vi "AplyDAQpars1.vi"(5 "AcqTimeIn":dbl) -> (1 "t1-t0":dbl, 3 "Idxs":i32[](array[numeric]))   [LabVIEW 2010]
uses:
  70user.lib/TheSigTab.vi
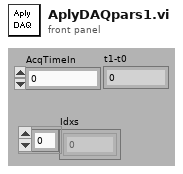
[diagram p1: front panel]
types:
  T1 = cluster{"Status":bool, "ViErrorNumber":u32, "ViName":string, "ViErrorString":string, "CinName":string, "CinErrorString":string}
  T2 = cluster{"s_Type":u16, "FIFO":u16, "IrqStep":u16, "Pages":u16, "AutoInit":u16, "dRate":dbl, "dKadr":dbl, "dScale":dbl, "Rate":u16, "Kadr":u16, "Scale":u16, "FPDelay":u16, "SynchroType":u16, "SynchroSensitivity":u16, "SynchroMode":u16, "AdChannel":u16, "AdPorog":u16, "NCh":u16, "Chn":i32[], "IrqEna":u16, "AdcEna":u16}
  T3 = cluster{"DllVersion":u32, "InterfaceType":u32, "InterfaceInstance":u32, "ModuleHandle":u32, "ReadBuffersParsArray":cluster{"Buffer":i16[], "ReadOv":u32, "ReadEvent":u32}[], "WriteBuffersParsArray":cluster{"Buffer":i16[], "WriteOv":u32, "WriteEvent":u32}[]}
  T4 = cluster{"VirtualSlot":u16, "ModuleName":string, "SerialNumber":string, "UsbSpeed":u8, "AvrVersion":string, "ModuleRevision":string, "DspType":string, "IsDacPresented":bool, "DspLoading":bool, "DspVersion":string, "DspClockout":u32, "AdcOffsetCoef":sgl[], "AdcScaleCoef":sgl[], "DacOffsetCoef":sgl[], "DacScaleCoef":sgl[]}
  T5 = cluster{"size":u16, "InputEnabled":bool, "CorrectionEnabled":bool, "InputClockSource":u16, "InputType":u16, "SynchroType":u16, "SynchroAdType":u16, "SynchroAdMode":u16, "SynchroAdChannel":u16, "SynchroAdPorog":i16, "ChannelsQuantity":u16, "ControlTable":u16[], "InputFifoBaseAddress":u16, "InputFifoLength":u16, "InputRate":dbl, "InterKadrDelay":dbl, "ChannelRate":dbl, "AdcOffsetCoefArray":dbl[], "AdcScaleCoefArray":dbl[], "BuffersLengthArray":u32[]}
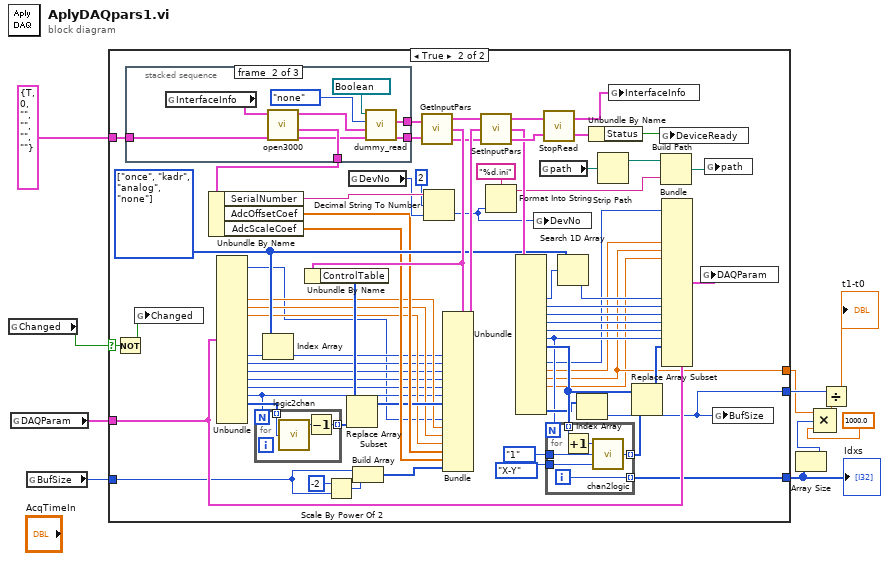
[diagram p0: block diagram]
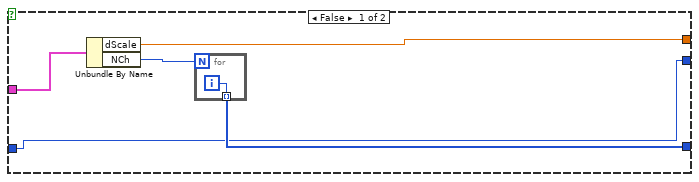
[diagram p2: hidden frame]
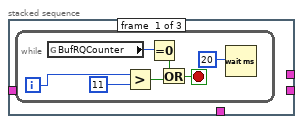
[diagram p3: hidden frame]
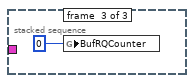
[diagram p4: hidden frame]
diagram:
  n1 = global read "TheSigTab.vi" "Changed"() -> (w11:bool)
  n2 = global read "TheSigTab.vi" "DAQParam"() -> (w10:T2)
  n3 = global read "TheSigTab.vi" "BufSize"() -> (w8:u32)
  n4 = case shown="True" w11 {
    selector: w11 -> [_ w66]
    tunnel: [w14 w46] -> w7
    tunnel: w10 -> [w16 w64]
    tunnel: T1 {"Status"=TRUE, "ViErrorNumber"=0, "ViName"="", "ViErrorString"="", "CinName"="", "CinErrorString"=""} ("ViStatusOut") -> [_ w60]
    tunnel: w8 -> [w12 w45]
    tunnel: [w12 w44] -> w6
    tunnel: [w13 w19] -> w5
    frame False {
      n5 = Unbundle By Name(w16) -> ("dScale"=w13:dbl, "NCh"=w15:u16)
      n6 = for {
        N: w15 -> [_]
        tunnel: [w17] -> w14 mode=indexing
        i -> [w17]
      }
    }
    frame True {
      w69 = enum16{"none", "once", "kadr", "analog"}[] [enum."once", enum."kadr", enum."analog", enum."none"] items=["none", "once", "kadr", "analog"]
      n7 = Not(x=w66) -> (.not. x?=w65:bool)
      n8 = stacked-sequence {
        tunnel: w60 -> [_ w101 _]
        tunnel: [_ w95 _] -> w59
        tunnel: [_ w96 _] -> w58
        tunnel: [_ w99 _] -> w57
        frame #0 {
          n9 = while {
            i -> [w91]
            stop <- w87 stop-if-true
            n10 = global read "TheSigTab.vi" "BufRQCounter"() -> (w92:i32)
            n11 = Greater?(x=w91, y=11) -> (0:w89:bool)
            n12 = Equal To 0?(x=w92) -> (x = 0?=w88:bool)
            n13 = Or(x=w88, y=w89) -> (x .or. y?=w87:bool)
            n14 = Wait (ms)(milliseconds to wait=u32 20) -> ()  [unwired: 1 out]
          }
        }
        frame #1 {
          n15 = global read "TheSigTab.vi" "InterfaceInfo"() -> (w100:T3)
          n16 = call "open3000.vi"("ViInfo"=w101, "InterfaceInfo"=w100) -> ("ViInfoOut"=w98:T1, "ModuleInfo"=w99:T4, "InterfaceInfoOut"=w97:T3)  [unwired: 3 in]
          n17 = call "dummy_read.vi"("ViStatusOut 2"=w98, "InterfaceInfoOut 2"=w97, "SyncType3000"=enum16{"none", "TTL", "TTL_kadr", "analog"}."none", "Ctrl Reference"=refnum<vi> refnum) -> ("ViStatusOut"=w96:T1, "InterfaceInfoOut"=w95:T3)  [unwired: 2 in]
        }
        frame #2 {
          n18 = global write "TheSigTab.vi" "BufRQCounter"(0 ("BufRQCounter")) -> ()
        }
      }
      n19 = global write "TheSigTab.vi" "Changed"(w65) -> ()
      n20 = Unbundle By Name(w57) -> ("SerialNumber"=w56:string, "AdcOffsetCoef"=w41:sgl[], "AdcScaleCoef"=w42:sgl[])
      n21 = Unbundle(w64) -> ("FIFO"=w22:u16, "dRate"=w37:dbl, "dKadr"=w36:dbl, "dScale"=w35:dbl, "SynchroType"=w71:u16, "SynchroSensitivity"=w30:u16, "SynchroMode"=w33:u16, "AdChannel"=w32:u16, "AdPorog"=w31:u16, "NCh"=w29:u16, "Chn"=w75:i32[])  [unwired: 10 out]
      n22 = for {
        N: w29 -> [_]
        tunnel: w75 -> [w111] mode=indexing
        tunnel: [w109] -> w83 mode=indexing
        n23 = call "logic2chan.vi"("value"=w111) -> ("Канал"=w110:u8)  [unwired: 2 out]
        n24 = Decrement(x=w110) -> (x-1=w109:u8)
      }
      n25 = Index Array(array=w69, index=w71) -> (element=w34:enum16{"none", "once", "kadr", "analog"})
      n26 = Scale By Power Of 2(n=-2, x=w45) -> (x*2^n=w68:u32)
      n27 = global read "TheSigTab.vi" "DevNo"() -> (w54:u32)
      n28 = Build Array(w45, w68) -> (w43:u32[])
      n29 = call "GetInputPars.vi"("InterfaceInfoIn"=w59, "ViStatusIn"=w58) -> ("InterfaceInfoOut"=w84:T3, "InputParsOut"=w74:T5, "ViStatusOut"=w63:T1)
      n30 = Unbundle By Name(w74) -> ("ControlTable"=w73:u16[])
      n31 = Replace Array Subset(array=w73, new element=w83) -> (w40:u16[])  [unwired: 1 in]
      n32 = Decimal String To Number(string=w56, offset=u32 2 ("initial scan location"), default (0L)=w54) -> (number=w47:u32)  [unwired: 1 out]
      n33 = Bundle(cluster=w74, "SynchroType"=w34, "SynchroAdType"=w30, "SynchroAdMode"=w33, "SynchroAdChannel"=w32, "SynchroAdPorog"=w31, "ChannelsQuantity"=w29, "ControlTable"=w40, "InputFifoLength"=w22, "InputRate"=w37, "InterKadrDelay"=w36, "ChannelRate"=w35, "AdcOffsetCoefArray"=w41, "AdcScaleCoefArray"=w42, "BuffersLengthArray"=w43) -> (w85:T5)  [unwired: 6 in]
      n34 = call "SetInputPars.vi"("ViStatusIn"=w63, "InputParsIn"=w85, "InterfaceInfoIn"=w84) -> ("ViStatusOut"=w81:T1, "InputParsOut"=w80:T5, "InterfaceInfoOut"=w82:T3)
      n35 = Format Into String(format string="%d.ini", w47) -> (resulting string=w49:string)  [unwired: 2 in, 1 out]
      n36 = Unbundle(w80) -> ("SynchroType"=w28:u16, "SynchroAdType"=w27:u16, "SynchroAdMode"=w26:u16, "SynchroAdChannel"=w25:u16, "SynchroAdPorog"=w24:i16, "ChannelsQuantity"=w23:u16, "ControlTable"=w39:u16[], "InputFifoLength"=w21:u16, "InputRate"=w20:dbl, "InterKadrDelay"=w19:dbl, "ChannelRate"=w18:dbl, "BuffersLengthArray"=w38:u32[])  [unwired: 8 out]
      n37 = global write "TheSigTab.vi" "DevNo"(w47) -> ()
      n38 = global read "TheSigTab.vi" "path"() -> (w51:path)
      n39 = call "StopRead.vi"("ViStatusIn"=w81, "InterfaceInfoIn"=w82) -> ("ViStatusOut"=w62:T1, "InterfaceInfoOut"=w61:T3)
      n40 = for {
        N: w23 -> [_]
        tunnel: w39 -> [w108] mode=indexing
        tunnel: [w107] -> w77 mode=indexing
        tunnel: enum16{"1", "2", "4", "8"}."1" ("Усиление") -> [w106]
        tunnel: enum16{"X-Y", "На землю", "X", "Y"}."X-Y" ("Switch") -> [w105]
        tunnel: [w103] -> w46 mode=indexing
        i -> [w103]
        n41 = Increment(x=w108) -> (x+1=w104:u16)
        n42 = call "chan2logic.vi"("Switch"=w105, "Усиление"=w106, "Канал"=w104) -> ("default value"=w107:u32)
      }
      n43 = Search 1D Array(1D array=w69, element=w28) -> (index of element=w70:i32)  [unwired: 1 in]
      n44 = Index Array(array=w38) -> (element=w44:u32)  [unwired: 1 in]
      n45 = Unbundle By Name(w62) -> ("Status"=w53:bool)
      n46 = Strip Path(path=w51) -> (stripped path=w50:path)  [unwired: 1 out]
      n47 = global write "TheSigTab.vi" "InterfaceInfo"(w61) -> ()
      n48 = Replace Array Subset(array=w39, new element=w77) -> (w76:u16[])  [unwired: 1 in]
      n49 = global write "TheSigTab.vi" "DeviceReady"(w53) -> ()
      n50 = Build Path(base path=w50, name or relative path=w49) -> (appended path=w52:path)
      n51 = Bundle(cluster=w64, "FIFO"=w21, "dRate"=w20, "dKadr"=w19, "dScale"=w18, "SynchroType"=w70, "SynchroSensitivity"=w27, "SynchroMode"=w26, "AdChannel"=w25, "AdPorog"=w24, "NCh"=w23, "Chn"=w76) -> (w72:T2)  [unwired: 10 in]
      n52 = global write "TheSigTab.vi" "DAQParam"(w72) -> ()
      n53 = global write "TheSigTab.vi" "path"(w52) -> ()
      n54 = global write "TheSigTab.vi" "BufSize"(w44) -> ()
    }
  }
  "Idxs" <- w7
  n55 = Array Size(array=w7) -> (size(s)=w4:i32)
  n56 = Compound Arithmetic op=MULTIPLY(w5, w4, 1000.0 ("t1-t0")) -> (w3:dbl)
  n57 = Divide(x=w6, y=w3) -> (x/y=→"t1-t0":dbl)
